vi "LEIN CMD create ACTI_6 PassThrough.vi"(0 "SID":u8, 1 "LEIN Variation":T3=enum."LEIN63", 5 "LEIN ecapsulated data (header and data)":u8[](array[numeric]), 9 "Sub Timeout (ms)":u16, 11 "error in (no error)":errorcluster) -> (8 "CMD":T1={"SID"=0, "ANF"=FALSE, "CMD"=enum."TASK", "DATA"=[]}, 15 "error out":errorcluster)   [LabVIEW 2011]
uses:
  Defenitions/LEIN Structure variations.ctl
  Defenitions/LEIN CMD Cluster.ctl
  Defenitions/LEIN CMD List.ctl
panel:
  # "ACTI 1 is Pass Through\n\nThis sends a message containinge another encapsuylation packed message, for retransmission."
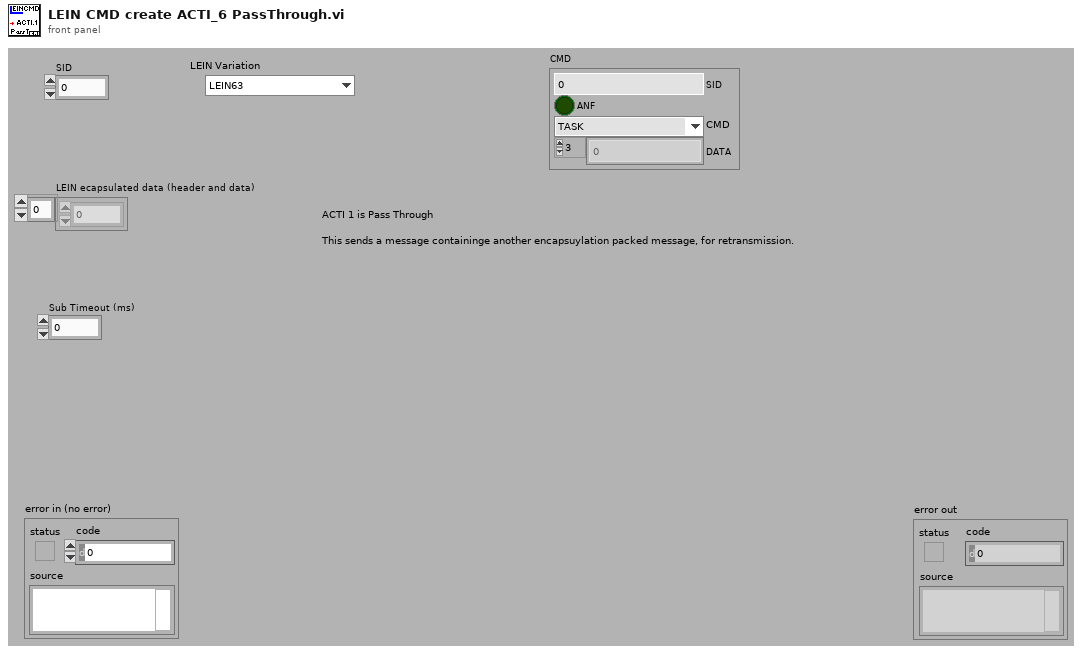
[diagram p1: front panel]
types:
  T1 = typedef "LEIN CMD Cluster.ctl" = cluster{"SID":u8, "ANF":bool, "CMD":T2, "DATA":u8[]}
  T2 = typedef "LEIN CMD List.ctl" = enum8{"ACTI", "TASK", "RES0", "STAT", "RES1", "RES2", "RES3", "USER"}
  T3 = typedef "LEIN Structure variations.ctl" = enum16{"LEIN08", "LEIN31", "LEIN63"}
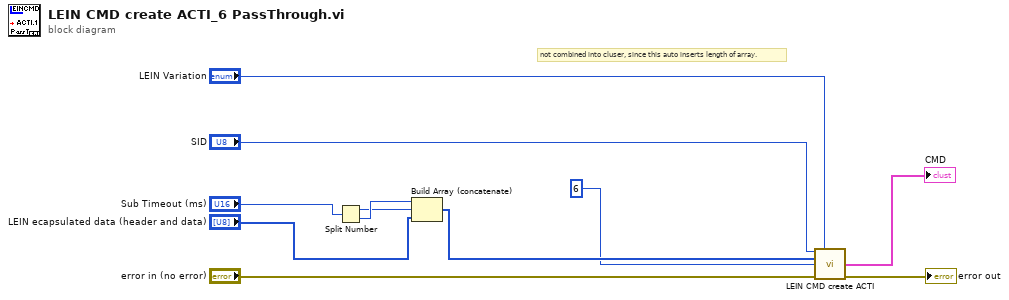
[diagram p0: block diagram]
diagram:
  # "not combined into cluser, since this auto inserts length of array."
  n1 = Split Number(x="Sub Timeout (ms)") -> (hi(x)=w6:u8, lo(x)=w7:u8)
  n2 = Build Array (concatenate)(w7, w6, "LEIN ecapsulated data (header and data)") -> (w4:u8[])
  n3 = call "LEIN CMD create ACTI.vi"("SID"="SID", "LEIN Variation"="LEIN Variation", "Data"=w4, "ACTI ID"=u8 6, "error in (no error)"="error in (no error)") -> ("CMD"=→"CMD":T1, "error out"=→"error out":errorcluster)  [unwired: 9 in]
